vi "Is Nested Runnable Active.vi"(10 "Name":string, 11 "Active Methods":set{string}(c389)) -> (3 "found?":bool)   [LabVIEW 2020, in "LUnit Test Suite.lvclass"]
uses:
  LUnit Test Suite.lvclass
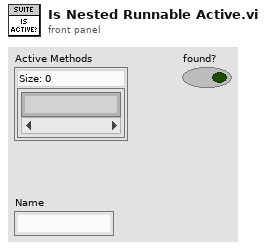
[diagram p1: front panel]
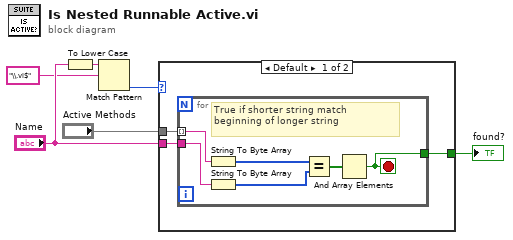
[diagram p0: block diagram]
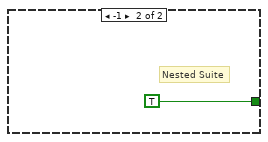
[diagram p2: hidden frame]
diagram:
  n1 = To Lower Case(string="Name") -> (all lower case string=w1:string)
  n2 = Match Pattern(string=w1, regular expression="\\.vi$") -> (offset past match=w2:i32)  [unwired: 1 in, 3 out]
  n3 = case shown="Default" w2 {
    tunnel: "Active Methods" -> [w9 _]
    tunnel: [w8 TRUE] -> w5
    tunnel: "Name" -> [w7 _]
    frame Default {
      n4 = for {
        tunnel: w9 -> [w15] mode=indexing
        tunnel: w7 -> [w14]
        tunnel: [w10] -> w8
        stop <- w10 stop-if-true
        # "True if shorter string match beginning of longer string"
        n5 = String To Byte Array(string=w15) -> (unsigned byte array=w13:u8[])
        n6 = String To Byte Array(string=w14) -> (unsigned byte array=w12:u8[])
        n7 = Equal?(x=w13, y=w12) -> (x = y?=w11:bool[])
        n8 = And Array Elements(Boolean array=w11) -> (logical AND=w10:bool)
      }
    }
    frame -1 {
      # "Nested Suite"
    }
  }
  "found?" <- w5
